vi "03. Native MQTT Service Client.vi"() -> ()   [LabVIEW 2019]
uses:
  Actor/Response -- cluster.ctl
  <vilib>/LabVIEW Open Source Project/MQTT Control Packets/Control Packets/ControlPacket/ControlPacket.lvclass/ControlPacket.ctl
  dd3c9ac1-01c7-4596-a0fc-d0451397087b.vi
  eb8eb180-2280-4b70-97f6-c873bf82b039.vi
  8ad8355e-0f22-4231-9c50-e2ed824064fe.vi
  b06ea2ed-6302-4e94-bd79-5b3576c24717.vi
  <vilib>/LabVIEW Open Source Project/MQTT Control Packets/Control Packets/PUBLISH/PUBLISH.lvclass
  C:/Program Files (x86)/National Instruments/LabVIEW 2019/vi.lib/LabVIEW Open Source Project/MQTT Control Packets/Control Packets/ControlPacket/ControlPacket.lvclass
  <vilib>/JDP Science/JSONtext/Variant to JSON Text.vi
  <vilib>/JDP Science/JSONtext/JSON text to Variant.vi
  <vilib>/JDP Science/JSONtext/LVClass Serializer/JSONtext LVClass Serializer.lvclass
  <vilib>/LabVIEW Open Source Project/MQTT Control Packets/Control Packets/ControlPacket/ControlPacket.lvclass
  <vilib>/JDP Science/JSONtext/JSONtext.lvlib
panel:
  out "methods":string[](array[string])
  out "ids":string[](array[string])
  out "Value":dbl
  out "Timestamp":timestamp
  in  "Service Namespace":string="demo/service"
  out "Topic":string
  out "<JSON>Response":string
  in  "parameters":string
  in  "Method":string
  in  "Send Req":bool
  in  "Get Value":bool
  in  "UTC?":bool
  in  "Get Timestamp":bool
  in  "Echo":bool
  # "Timeouts"
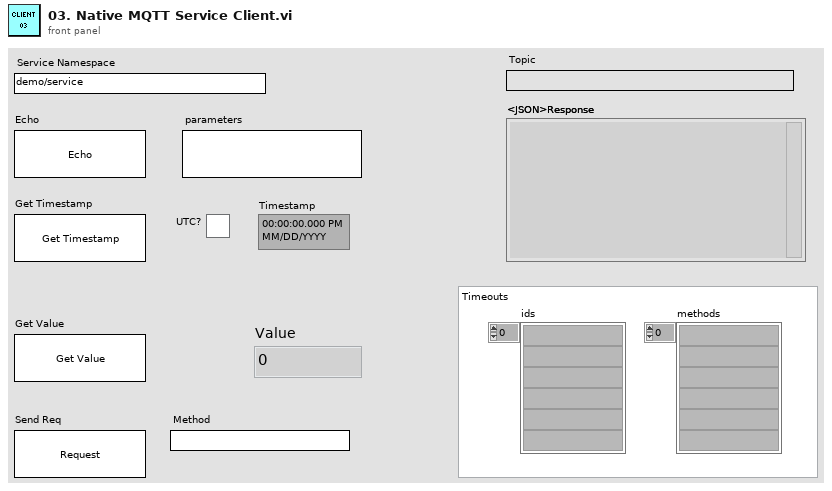
[diagram p1: front panel]
types:
  T1 = typedef "Actor Private Data.ctl" = cluster{"Client":refnum<class "Client.lvclass">, "QualifiedName":string, "EventReg":refnum<event-registration>, "Private Events":T2}
  T2 = typedef "Actor Private Events -- cluster.ctl" = cluster{"Stop":refnum<user-event>, "Subscribe":refnum<user-event>, "Unsubscribe":refnum<user-event>, "publish":refnum<user-event>}
  T3 = typedef "Response -- cluster.ctl" = cluster{"<JSON>result":string, "id":string, "<JSON>error":string}
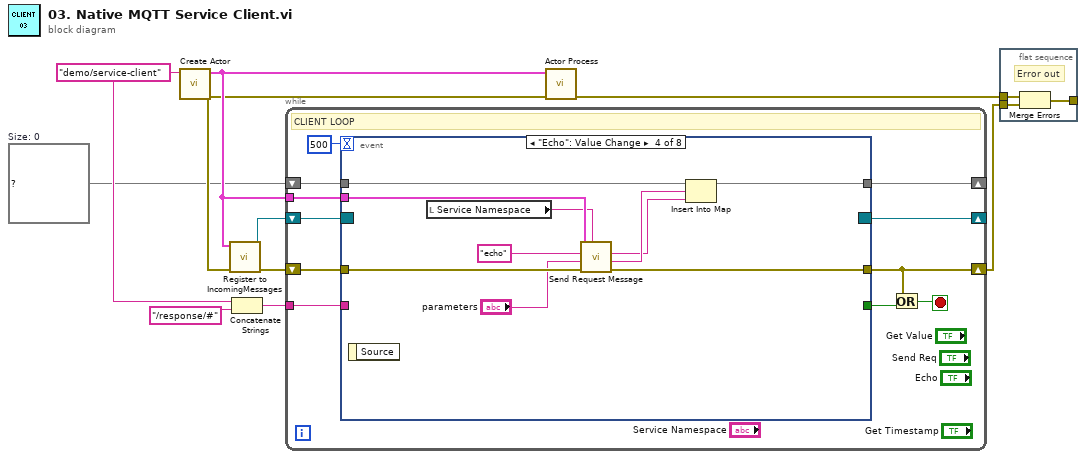
[diagram p0: block diagram]
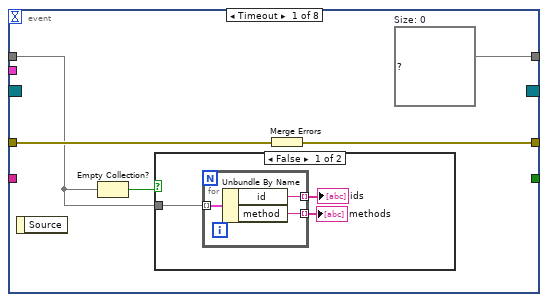
[diagram p2: hidden frame]
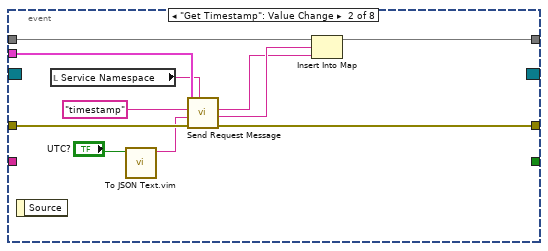
[diagram p4: hidden frame]
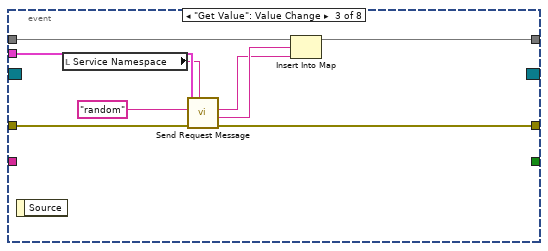
[diagram p5: hidden frame]
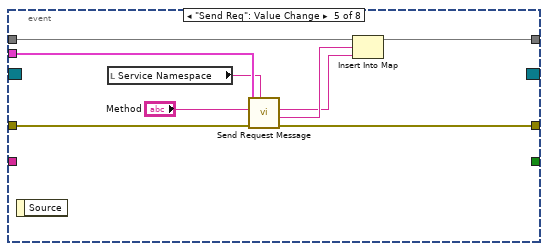
[diagram p6: hidden frame]
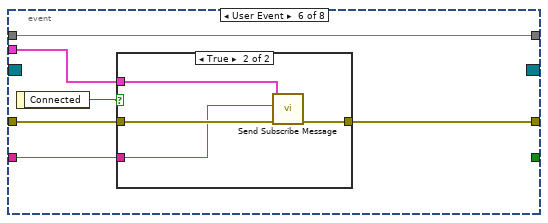
[diagram p7: hidden frame]
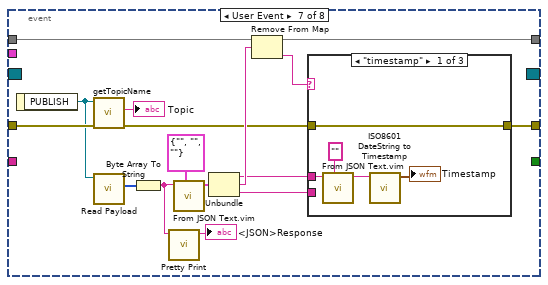
[diagram p9: hidden frame]
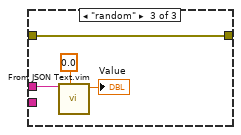
[diagram p11: hidden frame]
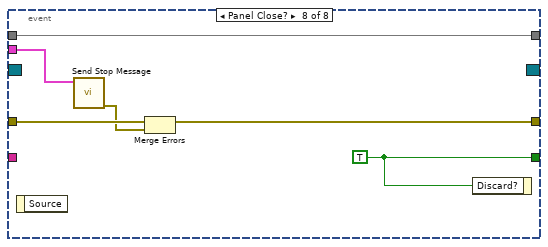
[diagram p12: hidden frame]
diagram:
  w1 = map{string, string} {}  # Size: 0
  w4 = "demo/service-client" ("QualifiedName")
  n1 = call "Create Actor.vi"("QualifiedName"=w4) -> ("error out"=w5:errorcluster, "Actor Class"=w9:T1)  [unwired: 9 in]
  n2 = call "Register to IncomingMessages.vi"("error in"=w5, "Actor Class"=w9) -> ("error out"=w8:errorcluster, "Incoming Messages"=w10:refnum<event-registration>)  [unwired: 8 in]
  n3 = Concatenate Strings(w4, "/response/#" ("QualifiedName")) -> (w2:string)
  n4 = while {
    tunnel: w9 -> [w19]
    shift-right: [w16] -> _
    shift-left: w10 -> [w17]
    shift-right: [w14] -> w7
    shift-left: w8 -> [w15]
    tunnel: w2 -> [w13]
    shift-right: [w11] -> _
    shift-left: w1 -> [w12]
    stop <- w20 stop-if-true
    # "CLIENT LOOP"
    n5 = event shown="[3] \"Echo\": Value Change" {
      selector: w17 -> [_ _ _ _ _ _ _ _]
      dyn-events: [_ _ _ _ _ _ _ _] -> w16
      timeout: 500 -> [_ _ _ _ _ _ _ _]
      tunnel: [_ _ _ _ _ _ _ w114] -> w21
      tunnel: w19 -> [_ w41 w50 w60 w69 w75 _ w113]
      tunnel: [w25 w42 w51 w61 w70 w76 w83 w110] -> w14
      tunnel: w15 -> [w26 w43 w52 w62 w71 w77 w98 w112]
      tunnel: w13 -> [_ _ _ _ _ w73 _ _]
      tunnel: w12 -> [w23 w38 w47 w56 w66 w72 w90 w109]
      tunnel: [w24 w35 w44 w53 w63 w72 w86 w109] -> w11
      event Timeout {
        w24 = map{string, string} {}  # Size: 0
        n6 = event-data() -> ()  [unwired: 1 in, 1 out]
        n7 = Empty Collection?(1:w23) -> (0:w22:bool)
        n8 = case shown="False" w22 {
          tunnel: w23 -> [w28 _]
          frame False {
            n9 = for {
              tunnel: w28 -> [w32] mode=indexing
              tunnel: [w31] -> w29 mode=indexing
              tunnel: [w30] -> w27 mode=indexing
              n10 = Unbundle By Name(w32) -> ("id"=w31:string, "method"=w30:string)
            }
            "ids" <- w29
            "methods" <- w27
          }
          frame True {
          }
        }
        n11 = Merge Errors(w26) -> (w25:errorcluster)
      }
      event "Get Timestamp": Value Change {
        n12 = event-data() -> ()  [unwired: 1 in, 1 out]
        n13 = local read "Service Namespace"() -> (w39:string)
        n14 = call "To JSON Text.vim"("Anything"="UTC?") -> ("<JSON>"=w33:string)  [unwired: 9 in, 1 out]
        n15 = call "Send Request Message.vi"("Qualified Name"=w39, "error in"=w43, "<JSON>params"=w33, "method"="timestamp", "Actor Class"=w41) -> ("error out"=w42:errorcluster, "id out"=w37:string, "method dup"=w36:string)  [unwired: 4 in]
        n16 = Insert Into Map(map in=w38, key=w37, value=w36) -> (map out=w35:map{string, string})  [unwired: 2 out]
      }
      event "Get Value": Value Change {
        n17 = event-data() -> ()  [unwired: 1 in, 1 out]
        n18 = local read "Service Namespace"() -> (w48:string)
        n19 = call "Send Request Message.vi"("Qualified Name"=w48, "error in"=w52, "method"="random", "Actor Class"=w50) -> ("error out"=w51:errorcluster, "id out"=w46:string, "method dup"=w45:string)  [unwired: 5 in]
        n20 = Insert Into Map(map in=w47, key=w46, value=w45) -> (map out=w44:map{string, string})  [unwired: 2 out]
      }
      event "Echo": Value Change {
        n21 = event-data() -> ()  [unwired: 1 in, 1 out]
        n22 = local read "Service Namespace"() -> (w57:string)
        n23 = call "Send Request Message.vi"("Qualified Name"=w57, "error in"=w62, "<JSON>params"="parameters", "method"="echo", "Actor Class"=w60) -> ("error out"=w61:errorcluster, "id out"=w55:string, "method dup"=w54:string)  [unwired: 4 in]
        n24 = Insert Into Map(map in=w56, key=w55, value=w54) -> (map out=w53:map{string, string})  [unwired: 2 out]
      }
      event "Send Req": Value Change {
        n25 = event-data() -> ()  [unwired: 1 in, 1 out]
        n26 = local read "Service Namespace"() -> (w67:string)
        n27 = call "Send Request Message.vi"("Qualified Name"=w67, "error in"=w71, "method"="Method", "Actor Class"=w69) -> ("error out"=w70:errorcluster, "id out"=w65:string, "method dup"=w64:string)  [unwired: 5 in]
        n28 = Insert Into Map(map in=w66, key=w65, value=w64) -> (map out=w63:map{string, string})  [unwired: 2 out]
      }
      event User Event {
        n29 = event-data() -> ("Connected"=w74:bool)  [unwired: 1 in]
        n30 = case shown="True" w74 {
          tunnel: w77 -> [w78 w82]
          tunnel: [w78 w81] -> w76
          tunnel: w75 -> [_ w80]
          tunnel: w73 -> [_ w79]
          frame False {
          }
          frame True {
            n31 = call "Send Subscribe Message.vi"("error in"=w82, "Topic"=w79, "Actor Class"=w80) -> ("error out"=w81:errorcluster)  [unwired: 8 in]
          }
        }
      }
      event User Event {
        n32 = event-data() -> ("PUBLISH"=w97:refnum<class "PUBLISH.lvclass">)  [unwired: 1 in]
        n33 = call <vilib>:"getTopicName.vi"("error in (no error)"=w98, "PUBLISH in"=w97) -> ("error out"=w84:errorcluster, "Topic"=→"Topic":string)  [unwired: 7 in, 1 out]
        n34 = call <vilib>:"Read Payload.vi"("ControlPacket in"=w97) -> ("Payload"=w96:u8[])  [unwired: 9 in, 1 out]
        n35 = Byte Array To String(unsigned byte array=w96) -> (string=w93:string)
        n36 = call <vilib>:"Pretty Print.vi"("JSON"=w93) -> ("<JSON>"=→"<JSON>Response":string)  [unwired: 8 in, 2 out]
        n37 = call "From JSON Text.vim"("Data Type and Default Value"=T3 {"<JSON>result"="", "id"="", "<JSON>error"=""} ("response"), "JSON"=w93) -> ("Data out"=w91:T3)  [unwired: 8 in, 1 out]
        n38 = Unbundle(w91) -> ("<JSON>result"=w88:string, "id"=w89:string, "<JSON>error"=w87:string)
        n39 = Remove From Map(10:w89, 11:w90) -> (1:w85:string, 3:w86:map{string, string})  [unwired: 1 out]
        n40 = case shown="\"timestamp\"" w85 {
          tunnel: w88 -> [w101 _ w106]
          tunnel: w87 -> [_ _ _]
          tunnel: w84 -> [w103 w104 w108]
          tunnel: [w103 w104 w108] -> w83
          frame "timestamp" {
            n41 = call "From JSON Text.vim"("Data Type and Default Value"="", "JSON"=w101) -> ("Data out"=w99:string)  [unwired: 8 in, 1 out]
            n42 = call <vilib>:"ISO8601 DateString to Timestamp.vi"("ISO8601 Date String"=w99) -> ("Timestamp"=→"Timestamp":timestamp)  [unwired: 8 in, 2 out]
          }
          frame Default {
          }
          frame "random" {
            n43 = call "From JSON Text.vim"("Data Type and Default Value"=0.0, "JSON"=w106) -> ("Data out"=→"Value":dbl)  [unwired: 8 in, 1 out]
          }
        }
      }
      event Panel Close? {
        w114 = TRUE ("Discard?")
        n44 = event-data() -> ()  [unwired: 1 in, 1 out]
        n45 = call "Send Stop Message.vi"("Actor Class"=w113) -> ("error out"=w111:errorcluster)  [unwired: 10 in]
        n46 = Merge Errors(w112, w111) -> (w110:errorcluster)
        n47 = event-data("Discard?"=w114) -> ()  [unwired: 1 in, 1 out]
      }
    }
    n48 = Or(x=w14, y=w21) -> (x .or. y?=w20:bool)
  }
  n49 = call "Actor Process.vi"("error in"=w5, "Actor Class"=w9) -> ("error out"=w6:errorcluster)  [unwired: 9 in]
  n50 = flat-sequence {
    tunnel: w6 -> [w117]
    tunnel: w7 -> [w116]
    tunnel: [w115] -> _
    frame #0 {
      # "Error out"
      n51 = Merge Errors(w117, w116) -> (w115:errorcluster)
    }
  }
